vi "load_data.vi"(0 "datasource_text_file in":refnum<class "datasource_text_file.lvclass">, 11 "error in (no error)":errorcluster) -> (4 "datasource_text_file out":refnum<class "datasource_text_file.lvclass">, 6 "document":refnum<class "data_document.lvclass">[](array[class]), 15 "error out":errorcluster)   [LabVIEW 2020, in "datasource_text_file.lvclass"]
uses:
  datasource_text_file.lvclass
  data/data_document/data_document.lvclass
  datasource_text_file.lvclass/datasource_text_file.ctl
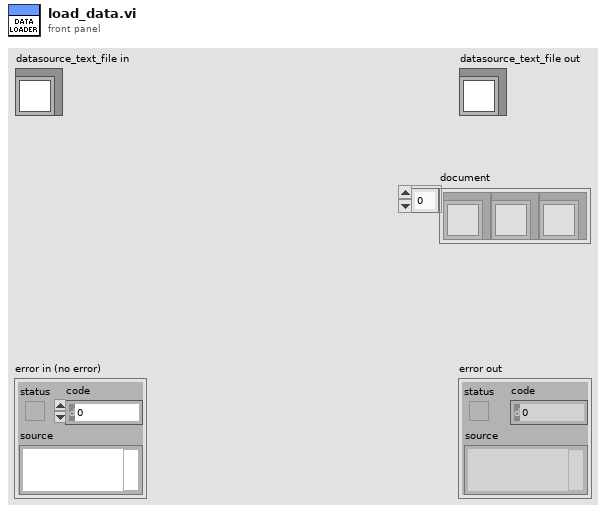
[diagram p1: front panel]
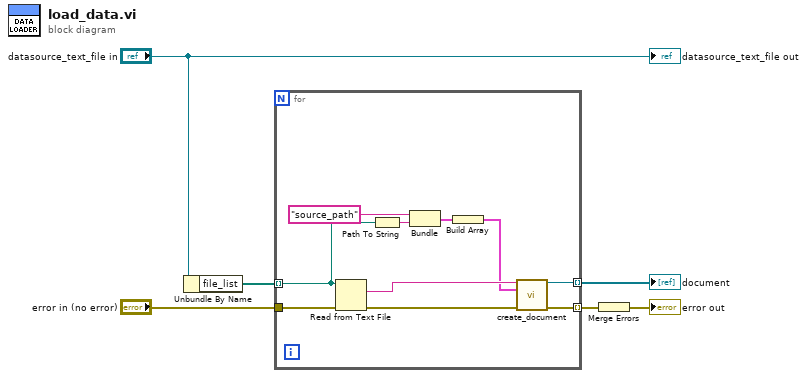
[diagram p0: block diagram]
diagram:
  n1 = Unbundle By Name("datasource_text_file in") -> ("file_list"=w5:path[])
  n2 = for {
    tunnel: w5 -> [w13] mode=indexing
    tunnel: "error in (no error)" -> [w16]
    tunnel: [w8] -> w3 mode=indexing
    tunnel: [w7] -> w1 mode=indexing
    n3 = Read from Text File(file (use dialog)=w13, error in=w16) -> (text=w15:string, error out=w9:errorcluster)  [unwired: 2 in, 2 out]
    n4 = Path To String(path=w13) -> (string=w12:string)
    n5 = Bundle("source_path", w12) -> (w11:cluster{string, string})  [unwired: 1 in]
    n6 = Build Array(w11) -> (w10:cluster{string, string}[])
    n7 = call "create_document.vi"("text"=w15, "metadatas"=w10, "error in (no error)"=w9) -> ("data_document out"=w7:refnum<class "data_document.lvclass">, "error out"=w8:errorcluster)  [unwired: 11 in]
  }
  "document" <- w1
  n8 = Merge Errors(w3) -> (→"error out":errorcluster)
  "datasource_text_file out" <- "datasource_text_file in"
